vi "Compute GB Size from directions.vi"() -> ()   [LabVIEW 2010]
panel:
  in  "Lattice Parameter":dbl
  out "appended array":dbl[](array[numeric])
  out "G2 Width Factor":dbl
  out "G1 Width Factor":dbl
  out "Near LCM height 'b'":dbl
  out "Near LCM viewing 'a'":dbl
  out "Lengths":dbl[](array[numeric])
  in  "Grain 2 Height ('b') 2":dbl[](array[numeric])=[1.0, 0.0, 0.0]
  in  "Grain 2 Viewing ('a') 2":dbl[](array[numeric])=[1.0, 0.0, 0.0]
  in  "Grain 2 Orientation ('c') 2":dbl[](array[numeric])=[1.0, 1.0, 1.0]
  in  "Grain 1 Height ('b')":dbl[](array[numeric])=[1.0, 0.0, 0.0]
  in  "Grain 1 Viewing ('a')":dbl[](array[numeric])=[1.0, 0.0, 0.0]
  in  "Tolerance":dbl
  in  "Grain 1 Orientation ('c')":dbl[](array[numeric])=[1.0, 1.0, 1.0]
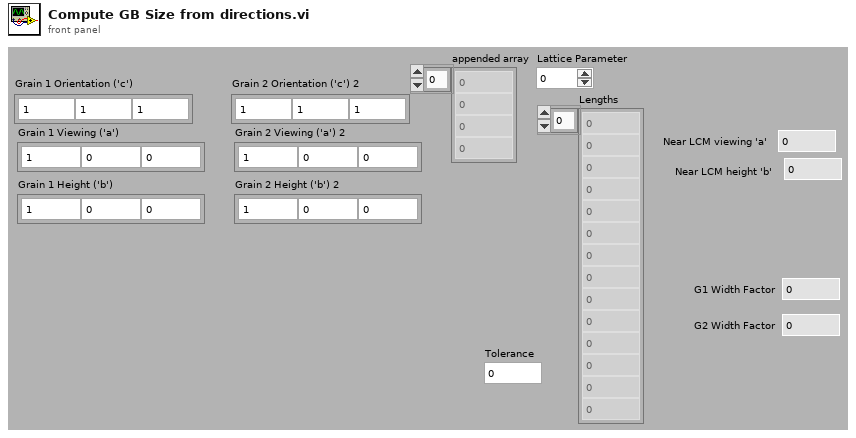
[diagram p1: front panel]
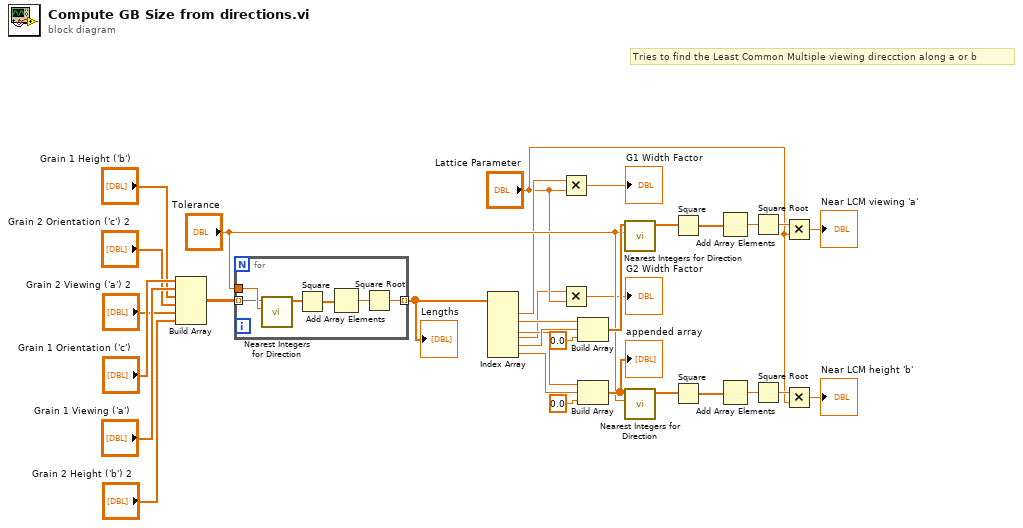
[diagram p0: block diagram]
diagram:
  # "Tries to find the Least Common Multiple viewing direcction along a or b"
  n1 = Build Array("Grain 1 Orientation ('c')", "Grain 1 Viewing ('a')", "Grain 1 Height ('b')", "Grain 2 Orientation ('c') 2", "Grain 2 Viewing ('a') 2", "Grain 2 Height ('b') 2") -> (w26:dbl[][])
  n2 = for {
    tunnel: [w35] -> w10 mode=indexing
    tunnel: "Tolerance" -> [w34]
    tunnel: w26 -> [w33] mode=indexing
    n3 = call "Nearest Integers for Direction.vi"("Tolerance"=w34, "Direction"=w33) -> ("Nearest Integer Directions"=w36:dbl[])  [unwired: 8 in, 1 out]
    n4 = Square(x=w36) -> (x^2=w37:dbl[])
    n5 = Add Array Elements(numeric array=w37) -> (sum=w38:dbl)
    n6 = Square Root(x=w38) -> (sqrt(x)=w35:dbl)
  }
  "Lengths" <- w10
  n7 = Index Array(array=w10) -> (element #1=w5:dbl, element #2=w23:dbl, element #3=w21:dbl, element #4=w2:dbl, element #5=w22:dbl, element #6=w20:dbl)  [unwired: 6 in]
  n8 = Multiply(x=w5, y="Lattice Parameter") -> (x*y=→"G1 Width Factor":dbl)
  n9 = Multiply(x=w2, y="Lattice Parameter") -> (x*y=→"G2 Width Factor":dbl)
  n10 = Build Array(w23, w22, 0.0 ("element")) -> (w19:dbl[])
  n11 = Build Array(w21, w20, 0.0 ("element")) -> (w18:dbl[])
  "appended array" <- w18
  n12 = call "Nearest Integers for Direction.vi"("Tolerance"="Tolerance", "Direction"=w19) -> ("Nearest Integer Directions"=w12:dbl[])  [unwired: 8 in, 1 out]
  n13 = call "Nearest Integers for Direction.vi"("Tolerance"="Tolerance", "Direction"=w18) -> ("Nearest Integer Directions"=w11:dbl[])  [unwired: 8 in, 1 out]
  n14 = Square(x=w12) -> (x^2=w16:dbl[])
  n15 = Square(x=w11) -> (x^2=w13:dbl[])
  n16 = Add Array Elements(numeric array=w16) -> (sum=w15:dbl)
  n17 = Add Array Elements(numeric array=w13) -> (sum=w14:dbl)
  n18 = Square Root(x=w15) -> (sqrt(x)=w7:dbl)
  n19 = Square Root(x=w14) -> (sqrt(x)=w9:dbl)
  n20 = Multiply(x=w7, y="Lattice Parameter") -> (x*y=→"Near LCM viewing 'a'":dbl)
  n21 = Multiply(x=w9, y="Lattice Parameter") -> (x*y=→"Near LCM height 'b'":dbl)
